vi "AutoRotate.vi"(8 "AccelRate":dbl, 9 "Actual":dbl, 10 "Desired":dbl) -> (2 "Right":dbl, 3 "Left":dbl)   [LabVIEW 2013]
doc: "The quickest and most efficient algorithm for automatically rotating the robot to a given orientation. Remember, winners us this VI."
uses:
  Robot Global Data.vi
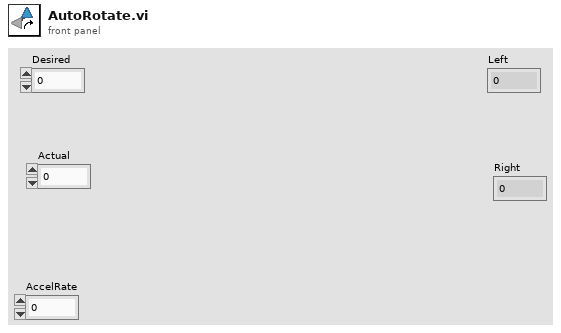
[diagram p1: front panel]
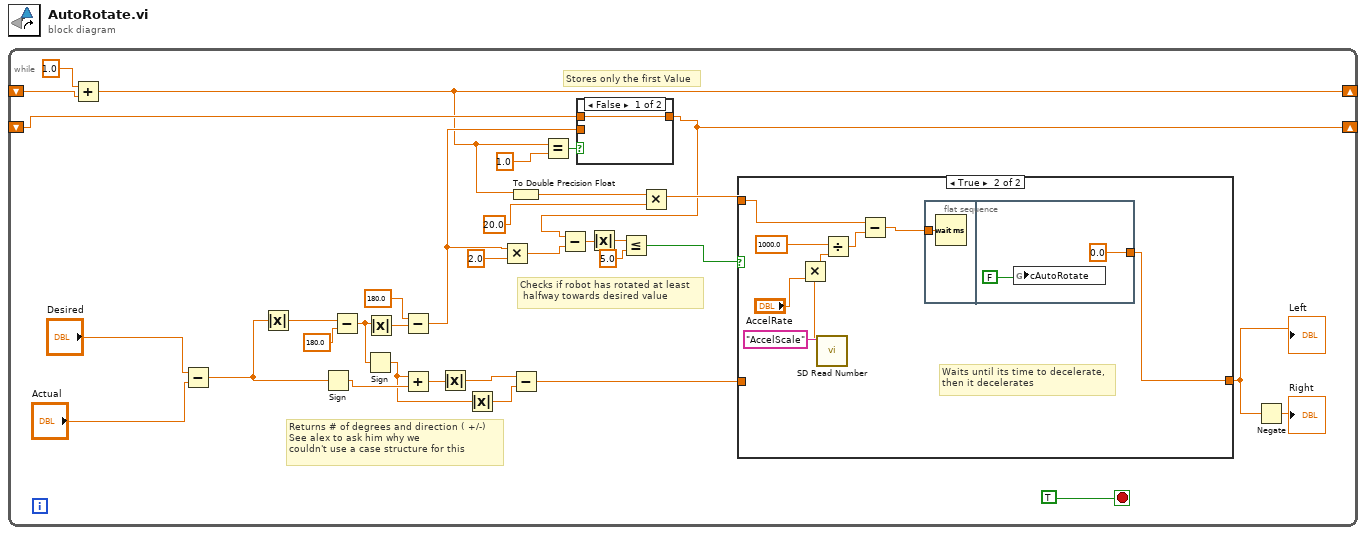
[diagram p0: block diagram]
diagram:
  n1 = while {
    shift-right: [w5] -> _
    shift-left: _ -> [w20]
    shift-right: [w8] -> _
    shift-left: _ -> [w9]
    stop <- TRUE stop-if-true
    # "Stores only the first Value"
    # "Checks if robot has rotated at least\n halfway towards desired value"
    # "Returns # of degrees and direction ( +/-)\nSee alex to ask him why we \ncouldn't use a case structure for this"
    n2 = Add(x=1.0, y=w9) -> (x+y=w8:dbl)
    n3 = Subtract(x="Desired", y="Actual") -> (x-y=w33:dbl)
    n4 = Absolute Value(x=w33) -> (abs(x)=w32:dbl)
    n5 = Sign(1:w33) -> (0:w17:dbl)
    n6 = Subtract(x=w32, y=180.0) -> (x-y=w27:dbl)
    n7 = Sign(1:w27) -> (0:w13:dbl)
    n8 = Absolute Value(x=w27) -> (abs(x)=w30:dbl)
    n9 = Subtract(x=180.0, y=w30) -> (x-y=w19:dbl)
    n10 = Add(x=w13, y=w17) -> (x+y=w16:dbl)
    n11 = Absolute Value(x=w16) -> (abs(x)=w15:dbl)
    n12 = Absolute Value(x=w13) -> (abs(x)=w14:dbl)
    n13 = Multiply(x=w19, y=2.0) -> (x*y=w4:dbl)
    n14 = To Double Precision Float(number=w8) -> (double precision float=w26:dbl)
    n15 = Subtract(x=w15, y=w14) -> (x-y=w12:dbl)
    n16 = Equal?(x=w8, y=1.0) -> (x = y?=w22:bool)
    n17 = case shown="False" w22 {
      tunnel: w19 -> [_ w36]
      tunnel: w20 -> [w35 _]
      tunnel: [w35 w36] -> w5
      frame False {
      }
      frame True {
      }
    }
    n18 = Subtract(x=w5, y=w4) -> (x-y=w3:dbl)
    n19 = Absolute Value(x=w3) -> (abs(x)=w1:dbl)
    n20 = Less Or Equal?(x=w1, y=5.0) -> (x <= y?=w21:bool)
    n21 = Multiply(x=w26, y=20.0) -> (x*y=w24:dbl)
    n22 = case shown="True" w21 {
      tunnel: [w37 w42] -> w6
      tunnel: w24 -> [_ w44]
      tunnel: w12 -> [w37 _]
      frame False {
      }
      frame True {
        # "Waits until its time to decelerate,\nthen it decelerates"
        n23 = call <vilib>:"SD Read Number.vi"("Name"="AccelScale") -> ("Numeric"=w40:dbl)  [unwired: 8 in, 2 out]
        n24 = Multiply(x="AccelRate", y=w40) -> (x*y=w38:dbl)
        n25 = Divide(x=1000.0, y=w38) -> (x/y=w45:dbl)
        n26 = Subtract(x=w44, y=w45) -> (x-y=w43:dbl)
        n27 = flat-sequence {
          tunnel: w43 -> [w47]
          tunnel: [0.0] -> w42
          frame #0 {
            n28 = Wait (ms)(milliseconds to wait=w47) -> ()  [unwired: 1 out]
          }
          frame #1 {
            n29 = global write "Robot Global Data.vi" "cAutoRotate"(FALSE) -> ()
          }
        }
      }
    }
    "Left" <- w6
    n30 = Negate(x=w6) -> (-x=→"Right":dbl)
  }
